vi "Teleop.vi"(10 "Match Info":T1={"Autonomous Elapsed Seconds"=0.0, "TeleOp Elapsed Seconds"=0.0, "Disabled Elapsed Seconds"=0.0, "Visited Autonomous"=FALSE, "Visited TeleOp"=FALSE, "Visited Disabled"=FALSE, "Autonomous Settings"={"Autonomous Style"=enum."Independent", "VI Refnum"=refnum}}, 11 "Call Context":T2) -> ()   [LabVIEW 2016]
doc: "This VI is called for each TeleOp packet received from the DS where the robot is not disabled. It is often used to read from the joysticks and update I/O or to update setpoints for timed control loops. It should complete and return within 20 milliseconds or it may miss DS packets."
uses:
  <vilib>/Rock Robotics/WPI/DriverStation/WPI_DriverStationDerivedRobotMode.ctl
  <vilib>/Rock Robotics/WPI/DriverStation/WPI_DriverStationMatch Info.ctl
  <vilib>/Rock Robotics/WPI/Utilities/WPI_GetSetVariantRefNum.vi
  Robot Global Data.vi
  <vilib>/Rock Robotics/Network Tables/NT Write Boolean Array.vi
  <vilib>/Rock Robotics/Network Tables/NT Write Numeric Array.vi
  <vilib>/Rock Robotics/Network Tables/NT Read Boolean.vi
  <vilib>/Rock Robotics/Network Tables/NT Read Number.vi
panel:
  out "Sample Slider 0":dbl(slide) scale=0.0..5.0
  out "Sample Boolean 1":bool
  out "Sample Boolean 0":bool
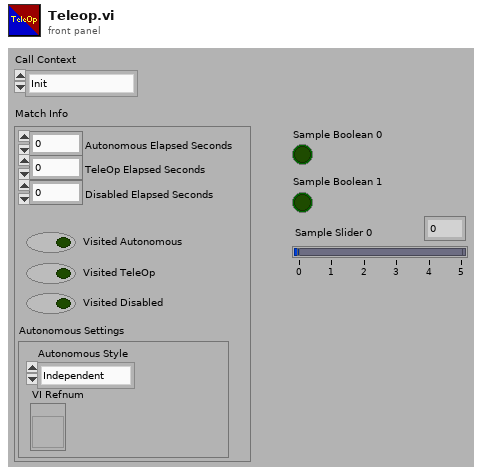
[diagram p1: front panel]
types:
  T1 = typedef "WPI_DriverStationMatch Info.ctl" = cluster{"Autonomous Elapsed Seconds":dbl, "TeleOp Elapsed Seconds":dbl, "Disabled Elapsed Seconds":dbl, "Visited Autonomous":bool, "Visited TeleOp":bool, "Visited Disabled":bool, "Autonomous Settings":cluster{"Autonomous Style":enum16{"Iterative", "Independent"}, "VI Refnum":refnum<vi>}}
  T2 = typedef "WPI_DriverStationDerivedRobotMode.ctl" = enum16{"Init", "Execute", "Stop"}
  T3 = typedef "WPI_JoystickDevRef.ctl" = cluster{"Device":T4}
  T4 = typedef "WPI_JoystickDeviceEnum.ctl" = enum16{"USB 0", "USB 1", "USB 2", "USB 3", "USB 4", "USB 5"}
  T5 = cluster{"Axes[0]":dbl, "Axes[1]":dbl, "Axes[2]":dbl, "Axes[3]":dbl, "Axes[4]":dbl, "Axes[5]":dbl, "Axes[6]":dbl, "Axes[7]":dbl, "Axes[8]":dbl}
  T6 = cluster{"Buttons[0]":bool, "Buttons[1]":bool, "Buttons[2]":bool, "Buttons[3]":bool, "Buttons[4]":bool, "Buttons[5]":bool, "Buttons[6]":bool, "Buttons[7]":bool, "Buttons[8]":bool, "Buttons[9]":bool}
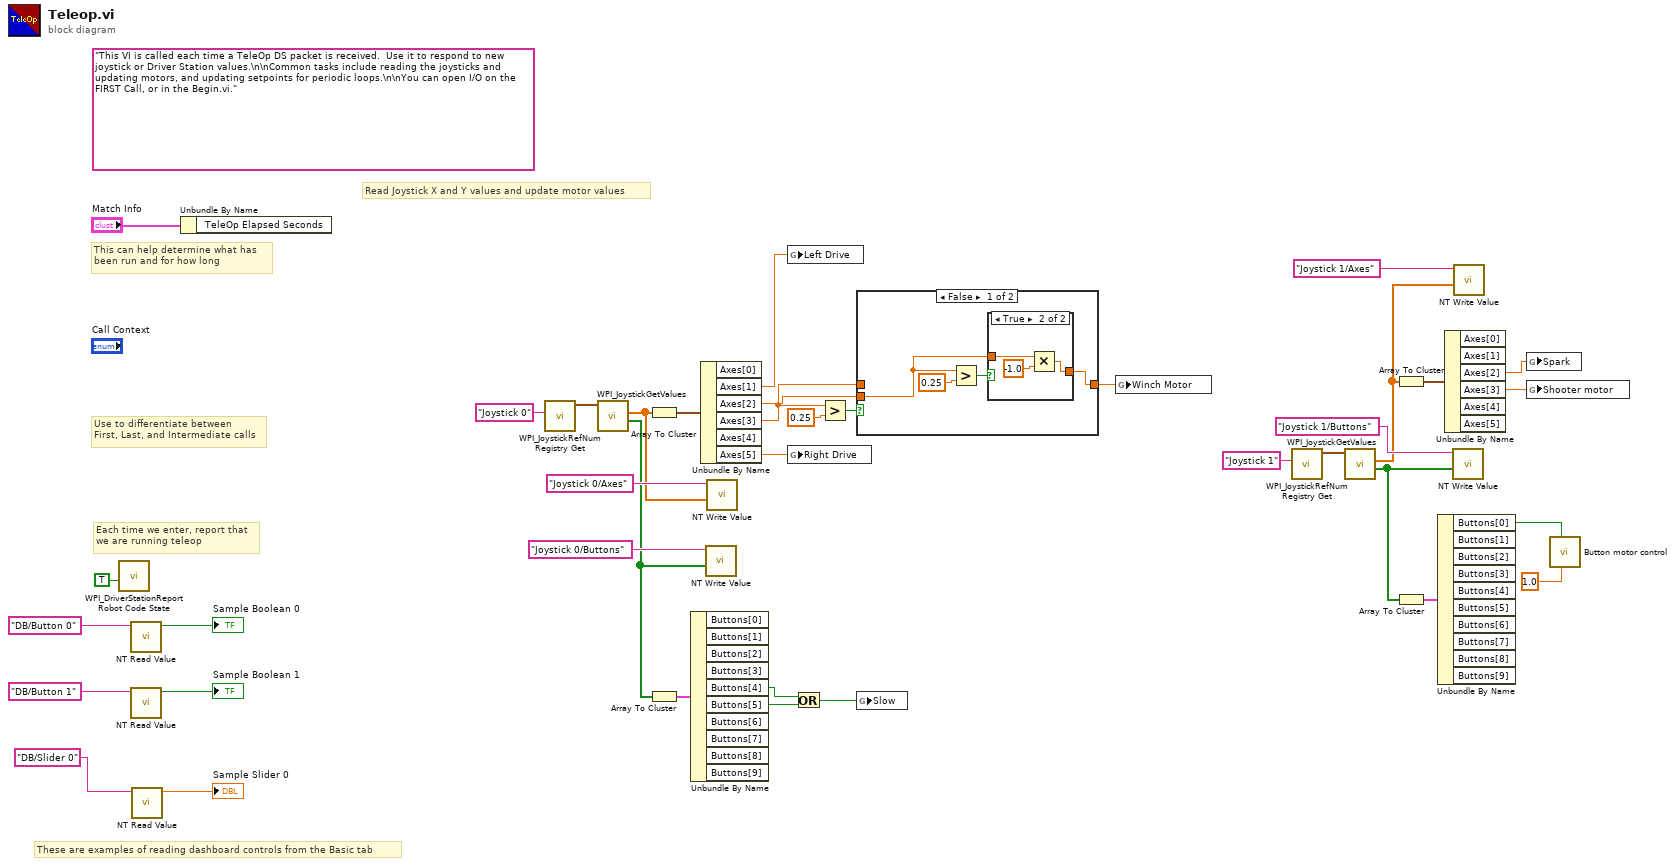
[diagram p0: block diagram]
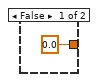
[diagram p2: hidden frame]
diagram:
  (unwired) "This VI is called each time a TeleOp DS packet is received.  Use it to respond to new joystick or Driver Station values.\n\nCommon tasks include reading the joysticks and updating motors, and updating setpoints for periodic loops.\n\nYou can open I/O on the FIRST Call, or in the Begin.vi."
  # "These are examples of reading dashboard controls from the Basic tab"
  # "Each time we enter, report that\nwe are running teleop"
  # "Use to differentiate between\nFirst, Last, and Intermediate calls"
  # "This can help determine what has\nbeen run and for how long"
  # "Read Joystick X and Y values and update motor values"
  n1 = call <vilib>:"WPI_DriverStationReport Robot Code State.vi"("TeleOp"=TRUE ("Autonomous")) -> ()  [unwired: 10 in, 1 out]
  n2 = call-poly <vilib>:"NT Read Value.vi"("Name"="DB/Button 0" ("refnum name")) -> ("Boolean"=→"Sample Boolean 0":bool)  [unwired: 9 in, 1 out]
  n3 = call-poly <vilib>:"NT Read Value.vi"("Name"="DB/Button 1" ("refnum name")) -> ("Boolean"=→"Sample Boolean 1":bool)  [unwired: 9 in, 1 out]
  n4 = call-poly <vilib>:"NT Read Value.vi"("Name"="DB/Slider 0" ("refnum name")) -> ("Numeric"=→"Sample Slider 0":dbl)  [unwired: 9 in, 1 out]
  n5 = Unbundle By Name("Match Info") -> ()  [unwired: 1 out]
  n6 = call <vilib>:"WPI_JoystickRefNum Registry Get.vi"("refnum name"="Joystick 0") -> ("JoystickDevRef"=w36:T3)  [unwired: 1 in, 9 out]
  n7 = call <vilib>:"WPI_JoystickGetValues.vi"("JoystickDevRef"=w36) -> ("Buttons"=w25:bool[], "Axes"=w26:dbl[])  [unwired: 6 in, 3 out]
  n8 = Array To Cluster(array=w26) -> (cluster=w23:T5)
  n9 = Array To Cluster(array=w25) -> (cluster=w24:T6)
  n10 = Unbundle By Name(w24) -> ("Buttons[4]"=w8:bool, "Buttons[5]"=w7:bool)  [unwired: 8 out]
  n11 = Unbundle By Name(w23) -> ("Axes[1]"=w21:dbl, "Axes[2]"=w1:dbl, "Axes[3]"=w3:dbl, "Axes[5]"=w22:dbl)  [unwired: 2 out]
  n12 = call-poly <vilib>:"NT Write Value.vi"("Boolean Array"=w25, "Name"="Joystick 0/Buttons") -> ()  [unwired: 9 in, 1 out]
  n13 = call-poly <vilib>:"NT Write Value.vi"("Numeric Array"=w26, "Name"="Joystick 0/Axes") -> ()  [unwired: 9 in, 1 out]
  n14 = global write "Robot Global Data.vi" "Left Drive"(w21) -> ()
  n15 = global write "Robot Global Data.vi" "Right Drive"(w22) -> ()
  n16 = Or(x=w8, y=w7) -> (x .or. y?=w6:bool)
  n17 = Greater?(x=w3, y=0.25) -> (0:w4:bool)
  n18 = case shown="False" w4 {
    tunnel: w3 -> [_ w47]
    tunnel: [w39 w47] -> w2
    tunnel: w1 -> [w40 _]
    frame False {
      n19 = Greater?(x=w40, y=0.25) -> (0:w41:bool)
      n20 = case shown="True" w41 {
        tunnel: w40 -> [_ w45]
        tunnel: [0.0 ("y") w44] -> w39
        frame False {
        }
        frame True {
          n21 = Multiply(x=w45, y=-1.0) -> (x*y=w44:dbl)
        }
      }
    }
    frame True {
    }
  }
  n22 = global write "Robot Global Data.vi" "Slow"(w6) -> ()
  n23 = global write "Robot Global Data.vi" "Winch Motor"(w2) -> ()
  n24 = call <vilib>:"WPI_JoystickRefNum Registry Get.vi"("refnum name"="Joystick 1") -> ("JoystickDevRef"=w19:T3)  [unwired: 1 in, 9 out]
  n25 = call <vilib>:"WPI_JoystickGetValues.vi"("JoystickDevRef"=w19) -> ("Buttons"=w15:bool[], "Axes"=w16:dbl[])  [unwired: 6 in, 3 out]
  n26 = Array To Cluster(array=w16) -> (cluster=w13:T5)
  n27 = Array To Cluster(array=w15) -> (cluster=w14:T6)
  n28 = Unbundle By Name(w14) -> ("Buttons[0]"=w10:bool)  [unwired: 9 out]
  n29 = Unbundle By Name(w13) -> ("Axes[2]"=w11:dbl, "Axes[3]"=w12:dbl)  [unwired: 4 out]
  n30 = call-poly <vilib>:"NT Write Value.vi"("Boolean Array"=w15, "Name"="Joystick 1/Buttons") -> ()  [unwired: 9 in, 1 out]
  n31 = call-poly <vilib>:"NT Write Value.vi"("Numeric Array"=w16, "Name"="Joystick 1/Axes") -> ()  [unwired: 9 in, 1 out]
  n32 = global write "Robot Global Data.vi" "Spark"(w11) -> ()
  n33 = global write "Robot Global Data.vi" "Shooter motor"(w12) -> ()
  n34 = call "Button motor control.vi"("Activate Button"=w10, "Requested Voltage %"=1.0) -> ()  [unwired: 9 in]
